vi "Setup.vi"(8 "error in (no error)":errorcluster, 11 "LUnit Test Runner Test In":refnum<class "Test Runner Test.lvclass">) -> (0 "error out":errorcluster, 3 "LUnit Test Runner Test Out":refnum<class "Test Runner Test.lvclass">)   [LabVIEW 2020, in "Test Runner Test.lvclass"]
doc: "Setup method called by the testing framework before each test method is called."
uses:
  Test Runner Test.lvclass
  Core/Result/Result.ctl
  Core/Result/Status.ctl
  Core/Result/Type.ctl
  Test Runner Test.lvclass/Test Runner Test.ctl
  Core/Result/Result.lvlib
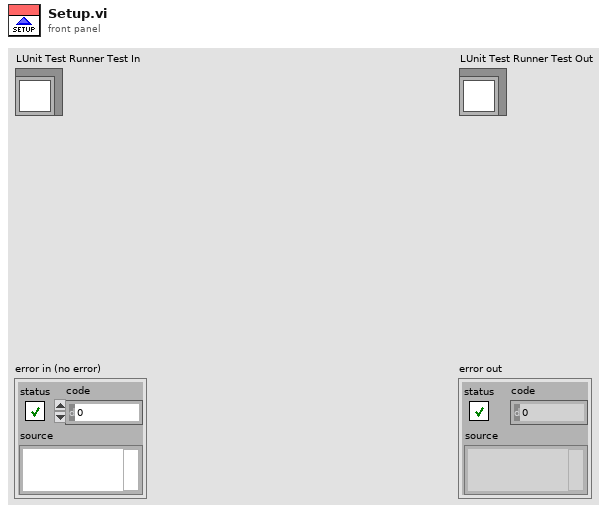
[diagram p1: front panel]
types:
  T1 = typedef "Result.lvlib/Result.ctl" = cluster{"Name":string, "Message":string, "Description":string, "Status":T2, "Result Type":T3, "Execution Time":dbl}
  T2 = typedef "Result.lvlib/Status.ctl" = enum16{"", "Passed", "Failed", "Error", "Skipped", "Setup Error", "Broken", "Teardown Error"}
  T3 = typedef "Result.lvlib/Type.ctl" = enum16{"Method", "Case", "Suite", "Pass", "Fail", "Skip", "Pass if", "Fail if", "Pass if Error", "Fail if Error", "Pass if Equal", "Fail if Equal"}
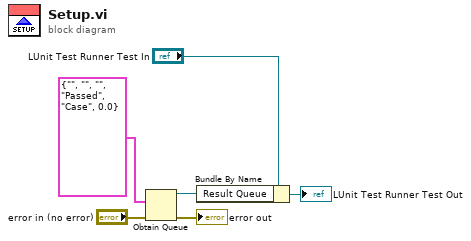
[diagram p0: block diagram]
diagram:
  n1 = Obtain Queue(element data type=T1 {"Name"="", "Message"="", "Description"="", "Status"=enum."Passed", "Result Type"=enum."Case", "Execution Time"=0.0} ("Result"), error in (no error)="error in (no error)") -> (queue out=w1:refnum<queue>, error out=→"error out":errorcluster)  [unwired: 3 in, 1 out]
  n2 = Bundle By Name(cluster="LUnit Test Runner Test In", "Result Queue"=w1) -> (→"LUnit Test Runner Test Out":refnum<class "Test Runner Test.lvclass">)
